vi "SCCAPI Get Project Name.vi"(8 "error in (no error)":errorcluster, 10 "configuration data":string) -> (0 "error out":errorcluster, 2 "project name":string)   [LabVIEW 2017, in "NI_SCC.lvlib"]
uses:
  <vilib>/SourceControl/sccapi/NI_SCC.lvlib
  <vilib>/SourceControl/sccapi/SCCAPI SCC Operations.ctl
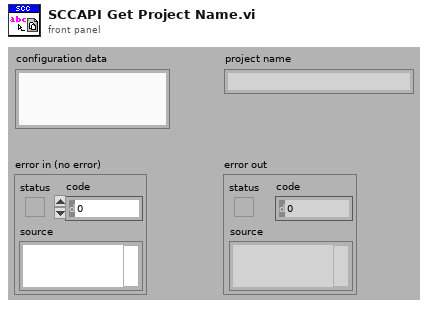
[diagram p1: front panel]
types:
  T1 = typedef "NI_SCC.lvlib/SCCAPI SCC Operations.ctl" = enum16{"Add", "Check In", "Check Out", "Close Project", "Compare Files", "Compare VIs", "Configure Project", "File History", "File Properties", "File Status", "Find All Providers", "Get Advanced Command Options", "Get File Copy", "Get Latest Version", "Get Project Name", "Get StaticVI Path", "Initialize", "Not A Source Control Reference", "Open Project", "Provider Supports Functionality", "Remove", "Run Provider", "Undo Check Out", "Uninitialize", "Is File In Local Path"}
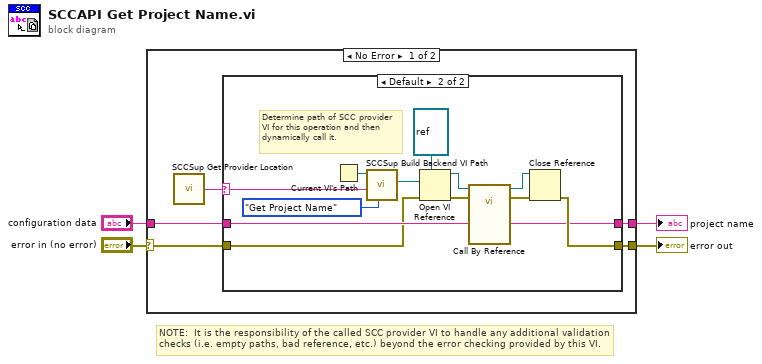
[diagram p0: block diagram]
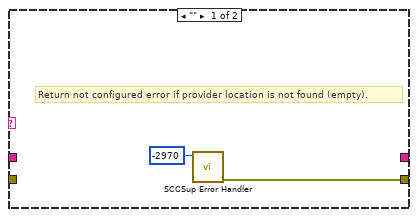
[diagram p2: hidden frame]
diagram:
  # "NOTE:  It is the responsibility of the called SCC provider VI to handle any additional validation checks (i.e. empty paths, bad reference, etc.) beyond the error checking provided by this VI."
  n1 = case shown="No Error" "error in (no error)" {
    selector: "error in (no error)" -> [w7 w25]
    tunnel: [w9 w25] -> w3
    tunnel: "configuration data" -> [w6 _]
    tunnel: [w5 _] -> w1
    frame No Error {
      n2 = call <vilib>:"SCCSup Get Provider Location.vi"() -> ("provider location"=w8:string)  [unwired: 6 in]
      n3 = case shown="Default" w8 {
        selector: w8 -> [_ w16]
        tunnel: [w10 w13] -> w9
        tunnel: w7 -> [_ w14]
        tunnel: w6 -> [_ w15]
        tunnel: [_ w12] -> w5
        frame "" {
          # "Return not configured error if provider location is not found (empty)."
          n4 = call <vilib>:"SCCSup Error Handler.vi"("scc error code"=-2970 ("code")) -> ("error out"=w10:errorcluster)  [unwired: 10 in]
        }
        frame Default {
          # "Determine path of SCC provider VI for this operation and then dynamically call it."
          n5 = Current VI's Path() -> (path=w23:path)
          n6 = call <vilib>:"SCCSup Build Backend VI Path.vi"("scc operation"=SCCAPI_SCC_Operations."Get Project Name", "provider location"=w16, "caller path"=w23) -> ("scc backend VI path"=w24:path)  [unwired: 8 in]
          n7 = Open VI Reference(type specifier VI Refnum (for type only)=refnum<vi> refnum, vi path=w24, error in (no error)=w14) -> (vi reference=w21:refnum<vi>, error out=w20:errorcluster)  [unwired: 3 in]
          n8 = call-by-ref "?"(reference=w21, error in=w20, "config data in"=w15) -> (reference out=w19:refnum<vi>, error out=w18:errorcluster, "project name"=w12:string)  [unwired: 8 in]
          n9 = Close Reference(reference=w19, error in (no error)=w18) -> (error out=w13:errorcluster)
        }
      }
    }
    frame Error {
    }
  }
  "error out" <- w3
  "project name" <- w1
